vi "UdsLogErrorCheckPoint.vi"(0 "UdsHandleIn":T1, 2 "LogSuspend":bool, 11 "error in":errorcluster) -> (4 "UdsHandleOut":T1, 15 "error out":errorcluster)   [LabVIEW 2011, in "Konvolucio MUDS150628.lvlib"]
uses:
  <instrlib>/Konvolucio MUDS150628/Konvolucio MUDS150628.lvlib
  <instrlib>/Konvolucio MUDS150628/Types/UdsHandleType.ctl
  <instrlib>/Konvolucio MCAN120803/Types/MCanHandleType.ctl
  C:/Program Files/National Instruments/LabVIEW 2011/instr.lib/Konvolucio MCAN120803/Private/Konvolucio.MCAN120803.dll
  Konvolucio MCAN120803/Private/Konvolucio.MCAN120803.dll
  <instrlib>/Konvolucio MCAN120803/Konvolucio MCAN120803.lvlib
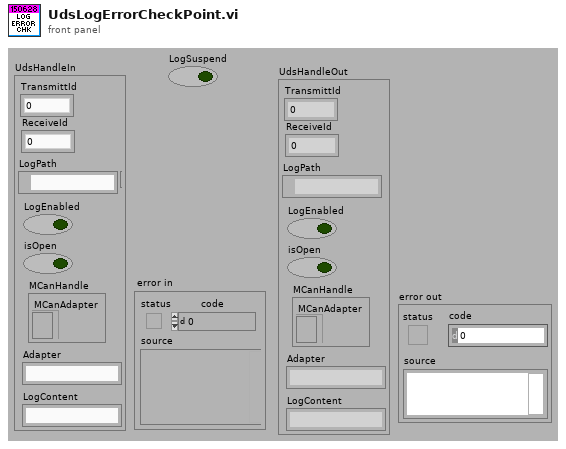
[diagram p1: front panel]
types:
  T1 = typedef "Konvolucio MUDS150628.lvlib/UdsHandleType.ctl" = cluster{"LogPath":path, "LogEnabled":bool, "isOpen":bool, "LogContent":string, "Adapter":string, "MCanHandle":T2, "TransmittId":u32, "ReceiveId":u32}
  T2 = typedef "Konvolucio MCAN120803.lvlib/MCanHandleType.ctl" = cluster{"MCanAdapter":refnum<k24>}
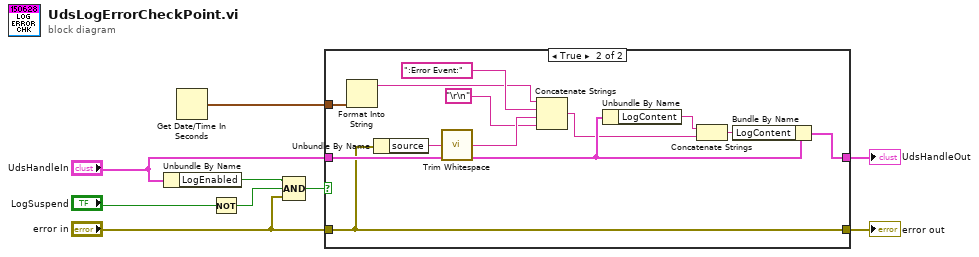
[diagram p0: block diagram]
diagram:
  n1 = Unbundle By Name("UdsHandleIn") -> ("LogEnabled"=w4:bool)
  n2 = Get Date/Time In Seconds() -> (seconds since 1Jan1904=w5:timestamp)
  n3 = Not(x="LogSuspend") -> (.not. x?=w2:bool)
  n4 = Compound Arithmetic op=AND(w4, w2, "error in") -> (w3:bool)
  n5 = case shown="True" w3 {
    tunnel: "error in" -> [w11 w12]
    tunnel: [w11 w12] -> w9
    tunnel: [w10 w23] -> w7
    tunnel: "UdsHandleIn" -> [w10 w22]
    tunnel: w5 -> [_ w19]
    frame False {
    }
    frame True {
      n6 = Format Into String(w19) -> (resulting string=w14:string)  [unwired: 3 in, 1 out]
      n7 = Unbundle By Name(w12) -> ("source"=w17:string)
      n8 = call <vilib>:"Trim Whitespace.vi"("string"=w17) -> ("trimmed string"=w18:string)  [unwired: 1 in]
      n9 = Concatenate Strings(w14, ":Error Event:" ("string"), w18, "\r\n") -> (w13:string)
      n10 = Unbundle By Name(w22) -> ("LogContent"=w20:string)
      n11 = Concatenate Strings(w20, w13) -> (w21:string)
      n12 = Bundle By Name(cluster=w22, "LogContent"=w21) -> (w23:T1)
    }
  }
  "error out" <- w9
  "UdsHandleOut" <- w7
